vi "T7 Stream Read KAG.vi"(0 "Connection ID In":refnum<k5>, 5 "IP Configuration":T1={"Connection ID In"=refnum, "Connection ID Out"=refnum, "Device IP"="192.168.126.147", "Port"=502}, 7 "Stream Configuration":T3={"Scan Rate (Hz)"=1000.0, "Samples Per Packet"=512, "Resolution Index"=0, "Buffer Size (bytes)"=32768, "NumScans"=1500, "Read Timeout (ms)"=5000.0, "Scan Table"=[{"Channel"=0, "BipGain"=0, "Input Config"="Single-Ended"}, {"Channel"=1, "BipGain"=0, "Input Config"="Single-Ended"}, {"Channel"=2, "BipGain"=0, "Input Config"="Single-Ended"}, {"Channel"=3, "BipGain"=0, "Input Config"="Single-Ended"}]} {"Samples Per Packet" max=512 step=1; "Buffer Size (bytes)" max=32768 step=1; "Resolution Index" max=8 step=1; "Scan Rate (Hz)" min=0.0 max=100000.0; "Scan Table"."BipGain" max=3 step=1; "Scan Table"."Channel" step=1}, 9 "Secondary Stream Configurations":T2={"Settling Delay (*5 us)"=0.0, "Clock Source"=0, "Auto Target"=1} {"Auto Target" max=255 step=1; "Clock Source" max=2 step=2; "Settling Delay (*5 us)" min=0.0 max=5000.0 step=1.0}, 11 "error in":errorcluster) -> (6 "Read Array":u8[](array[numeric]) format="%.0x", 8 "TCP Data":string, 15 "error out":errorcluster)   [LabVIEW 2015]
doc: "Read Stream Data at Ethernet Socket 702."
uses:
  T7 Stream Config KAG.ctl
  T7 Secondary Configs KAG.ctl
  T7 IP Config KAG.ctl
  T7 Stream Globals KAG.vi
panel:
  in  "Tab Control":enum32{"TCP Read Data"}(tab)
  out "# of bytes received":i32
  out "# Bytes to Read":i32
  out "Scan Interval":dbl
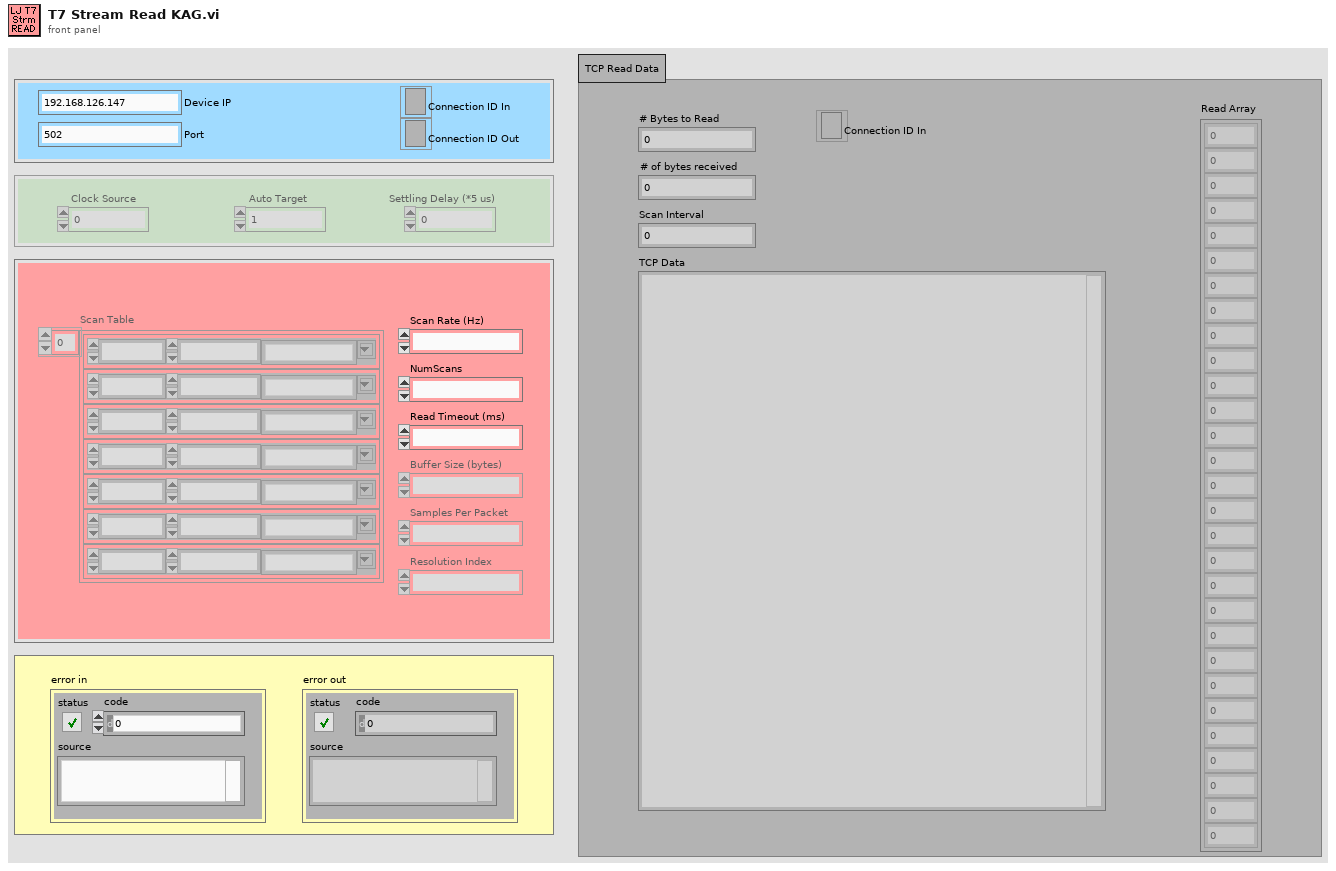
[diagram p1: front panel]
types:
  T1 = typedef "T7 IP Config KAG.ctl" = cluster{"Connection ID In":refnum<k5>, "Connection ID Out":refnum<k5>, "Device IP":string, "Port":i32}
  T2 = typedef "T7 Secondary Configs KAG.ctl" = cluster{"Settling Delay (*5 us)":dbl, "Clock Source":u32, "Auto Target":u32}
  T3 = typedef "T7 Stream Config KAG.ctl" = cluster{"Scan Rate (Hz)":dbl, "Samples Per Packet":u32, "Resolution Index":u32, "Buffer Size (bytes)":u32, "NumScans":u32, "Read Timeout (ms)":dbl, "Scan Table":cluster{"Channel":u32, "BipGain":u32, "Input Config":string}[]}
  T4 = cluster{"Channel":u32, "BipGain":u32, "Input Config":string}[]
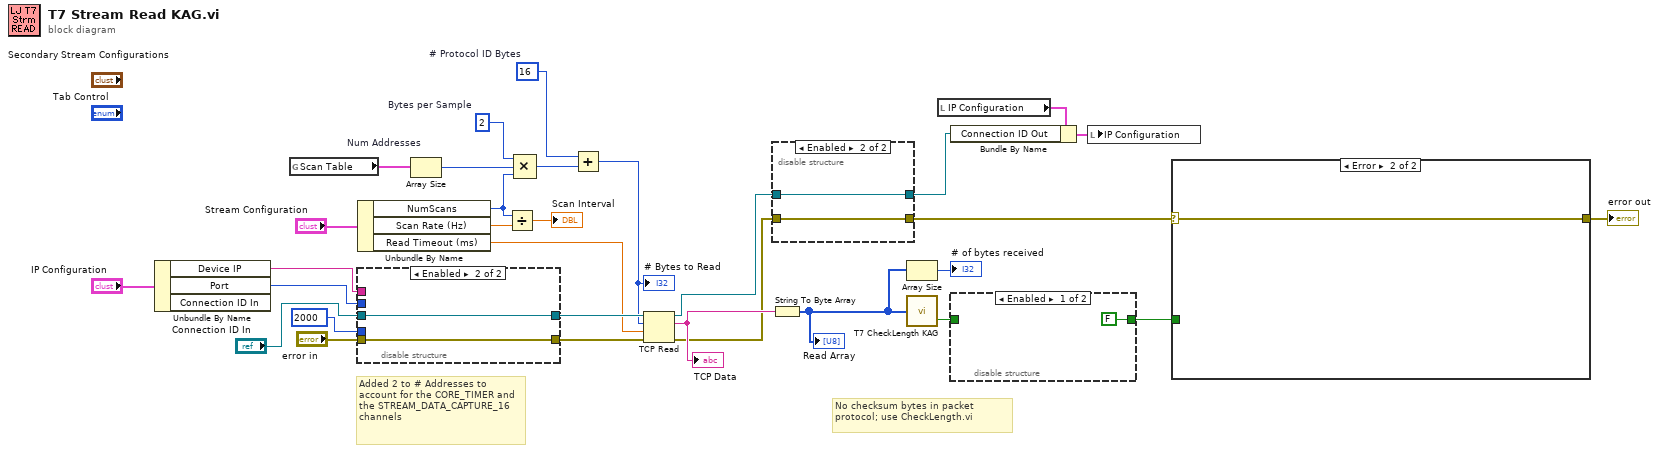
[diagram p0: block diagram]
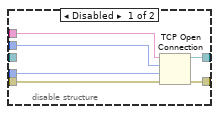
[diagram p2: hidden frame]
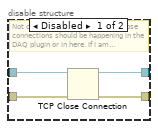
[diagram p4: hidden frame]
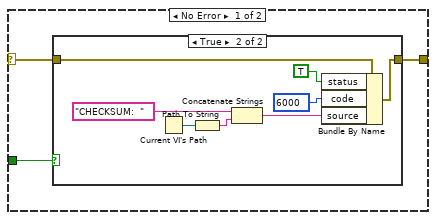
[diagram p5: hidden frame]
diagram:
  w18 = u32 16  # # Protocol ID Bytes
  w4 = 2  # Bytes per Sample
  # "Added 2 to # Addresses to account for the CORE_TIMER and the STREAM_DATA_CAPTURE_16 channels"
  # "No checksum bytes in packet protocol; use CheckLength.vi"
  n1 = Unbundle By Name("IP Configuration") -> ("Device IP"=w11:string, "Port"=w10:i32)  [unwired: 1 out]
  n2 = global read "T7 Stream Globals KAG.vi" "Scan Table"() -> (w21:T4)
  n3 = Unbundle By Name("Stream Configuration") -> ("NumScans"=w2:u32, "Scan Rate (Hz)"=w5:dbl, "Read Timeout (ms)"=w9:dbl)
  n4 = disable-structure shown="Enabled" {
    disable-tunnel: 2000 ("timeout ms (60000)") -> [w37 _]
    disable-tunnel: w11 -> [w36 _]
    disable-tunnel: "error in" -> [w35 w39]
    disable-tunnel: [w34 w39] -> w26
    disable-tunnel: [w33 w38] -> w25
    disable-tunnel: w10 -> [w32 _]
    disable-tunnel: "Connection ID In" -> [_ w38]
    frame Disabled {
      n5 = TCP Open Connection(address=w36, remote port or service name=w32, timeout ms (60000)=w37, error in (no error)=w35) -> (connection ID=w33:refnum<k5>, error out=w34:errorcluster)  [unwired: 1 out]
    }
    frame Enabled {
    }
  }
  n6 = Array Size "Num Addresses"(array=w21) -> (size(s)=w3:i32)
  n7 = Divide(x=w2, y=w5) -> (x/y=→"Scan Interval":dbl)
  n8 = Compound Arithmetic op=MULTIPLY(w4, w3, w2) -> (w22:u32)
  n9 = Add(x=w18, y=w22) -> (x+y=w17:u32)
  "# Bytes to Read" <- w17
  n10 = TCP Read(connection ID=w25, bytes to read=w17, error in (no error)=w26, 9:w9) -> (connection ID out=w16:refnum<k5>, data out=w30:string, error out=w15:errorcluster)  [unwired: 1 out]
  "TCP Data" <- w30
  n11 = String To Byte Array(string=w30) -> (unsigned byte array=w24:u8[])
  "Read Array" <- w24
  n12 = disable-structure shown="Enabled" {
    disable-tunnel: w16 -> [w43 w45]
    disable-tunnel: w15 -> [w42 w44]
    disable-tunnel: [w41 w45] -> w7
    disable-tunnel: [w40 w44] -> w14
    frame Disabled {
      # "Not clear whether the open and close connections should be happening in the DAQ plugin or in here. If I am recursively doing TCP reads, wouldn't make any sense to open and close tcp connection every time"
      n13 = TCP Close Connection(connection ID=w43, error in (no error)=w42) -> (connection ID out=w41:refnum<k5>, error out=w40:errorcluster)  [unwired: 1 in]
    }
    frame Enabled {
    }
  }
  n14 = Array Size(array=w24) -> (size(s)=→"# of bytes received":i32)
  n15 = call "T7 CheckLength KAG.vi"("Array"=w24) -> ("CheckLength Error"=w19:bool)  [unwired: 1 out]
  n16 = local read "IP Configuration"() -> (w8:T1)
  n17 = Bundle By Name(cluster=w8, "Connection ID Out"=w7) -> (w6:T1)
  n18 = disable-structure shown="Enabled" {
    disable-tunnel: [FALSE w47] -> w20
    disable-tunnel: w19 -> [_ w47]
    frame Enabled {
    }
    frame Disabled {
    }
  }
  n19 = local write "IP Configuration"(w6) -> ()
  n20 = case shown="Error" w14 {
    selector: w14 -> [w50 w60]
    tunnel: [w49 w60] -> w28
    tunnel: w20 -> [w48 _]
    frame No Error {
      n21 = case shown="True" w48 {
        tunnel: w50 -> [w51 w59]
        tunnel: [w51 w58] -> w49
        frame False {
        }
        frame True {
          n22 = Current VI's Path() -> (path=w56:path)
          n23 = Path To String(path=w56) -> (string=w54:string)
          n24 = Concatenate Strings("CHECKSUM:  " ("Substring"), w54) -> (w53:string)
          n25 = Bundle By Name(cluster=w59, "status"=TRUE, "code"=u32 6000 ("y"), "source"=w53) -> (w58:errorcluster)
        }
      }
    }
    frame Error {
    }
  }
  "error out" <- w28
